vi "AWGCompileContinuousWave.vi"(2 "error in":errorcluster, 3 "ArbitraryWaveListMW":dbl[][](array[numeric]) caption="Arbitrary Waveform List") -> (0 "error out":errorcluster, 1 "array MW and RF":variant[](array[variant]))   [LabVIEW 2019]
panel:
  out "AWG array out":variant[](array[variant])
  in  "Timing cluster 2":T1
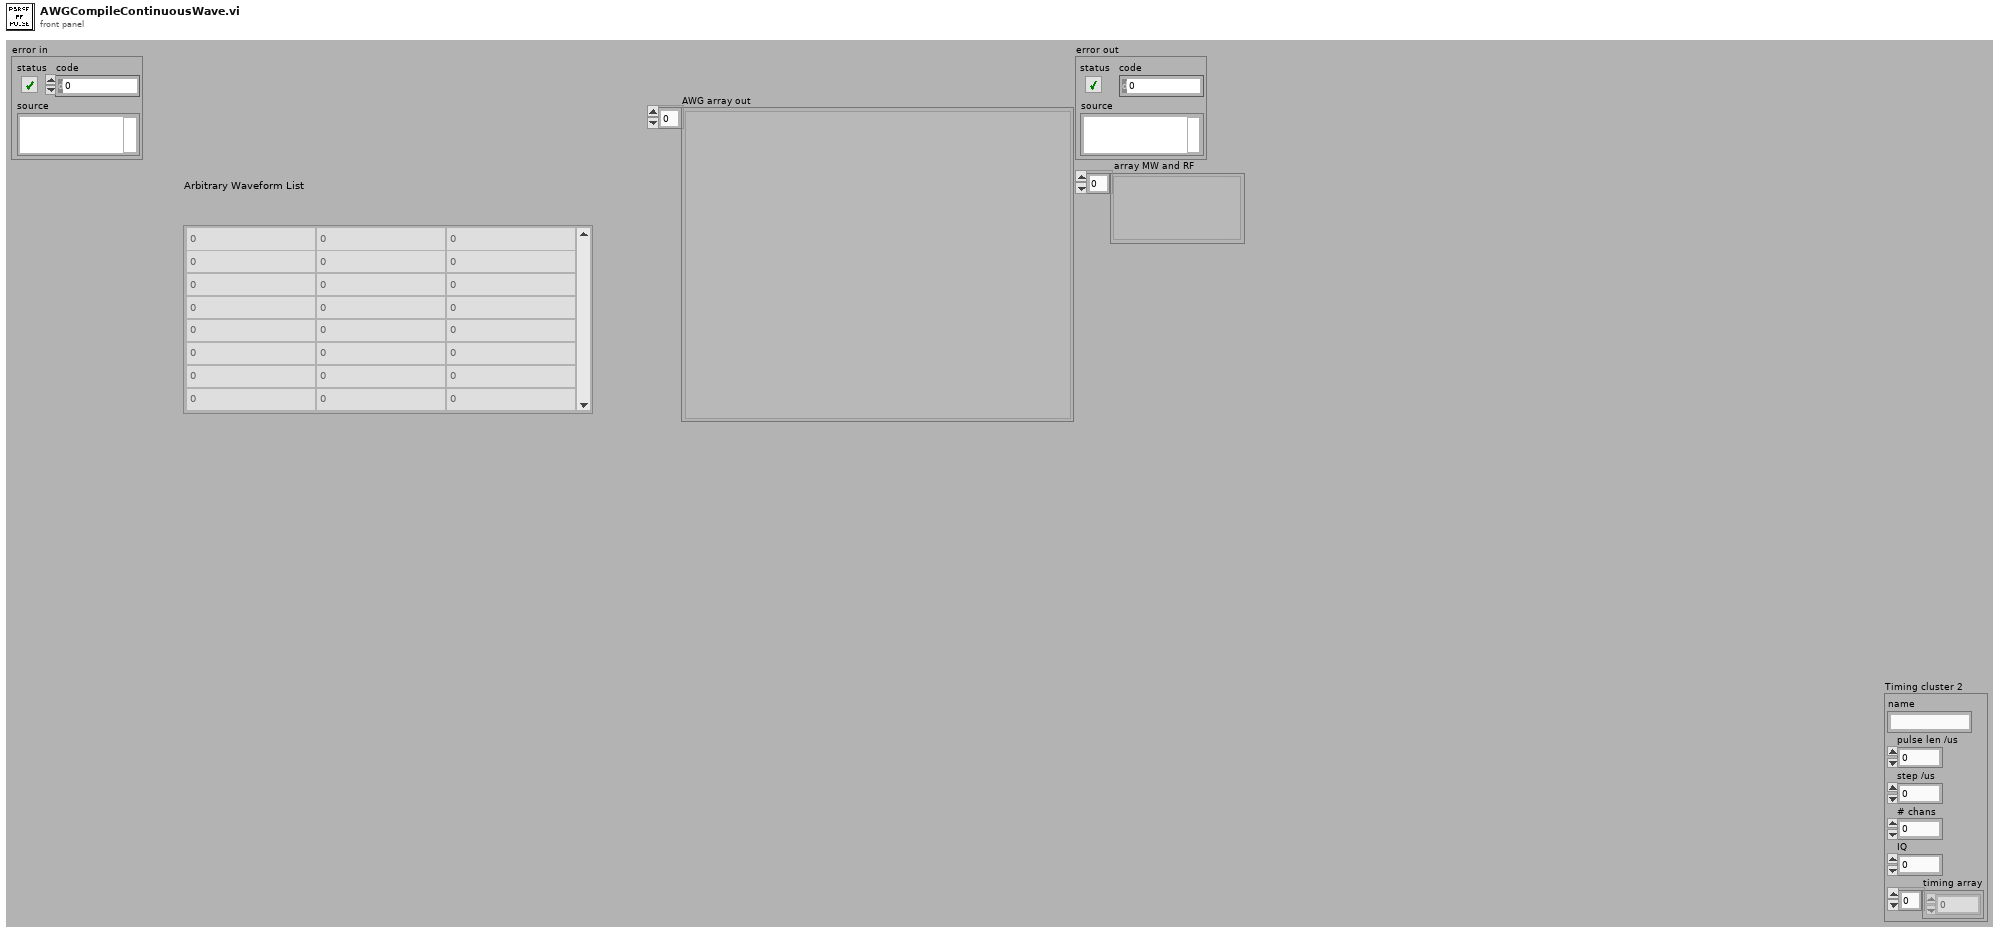
[diagram p1: front panel]
types:
  T1 = cluster{"name":string, "pulse len /us":dbl, "step /us":dbl, "# chans":i32, "IQ":i32, "timing array":dbl[]}
  T2 = cluster{"Timing cluster 2":cluster{"name":string, "pulse len /us":dbl, "step /us":dbl, "# chans":i32, "IQ":i32, "timing array":dbl[]}, "Channel cluster 2":cluster{"amp":dbl, "amp step":dbl, "channel array":dbl[]}[]}
  T3 = cluster{"amp":dbl, "amp step":dbl, "array type (2D Dbl)":dbl[]}
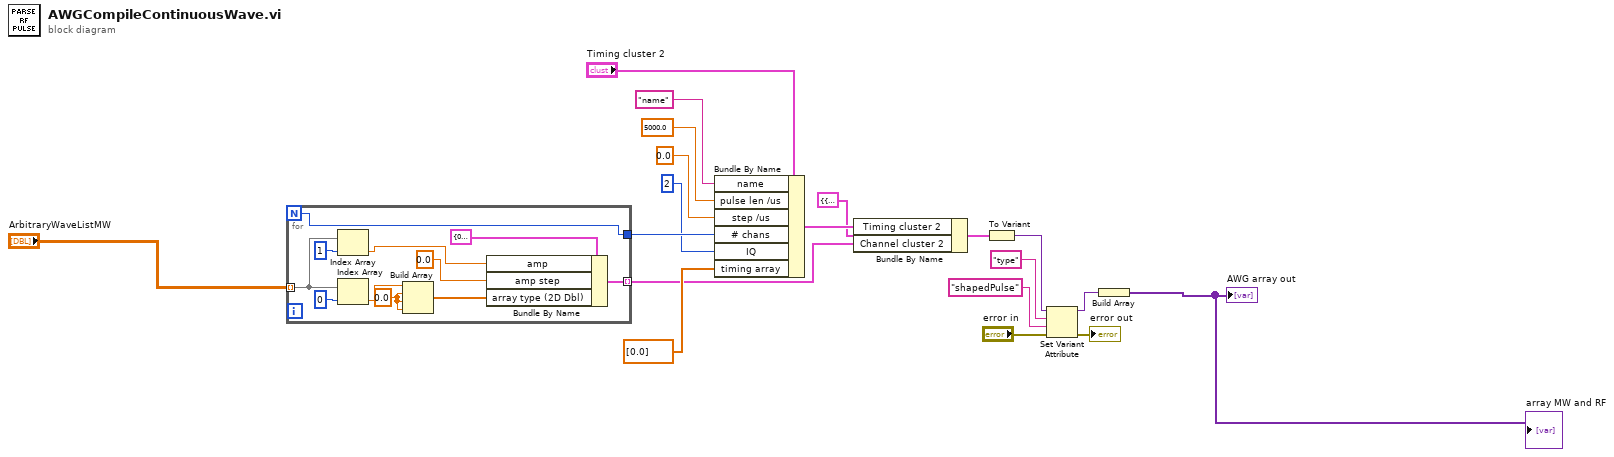
[diagram p0: block diagram]
diagram:
  n1 = for {
    N -> [w26]
    tunnel: "ArbitraryWaveListMW" -> [w23] mode=indexing
    tunnel: [w26] -> w9
    tunnel: [w20] -> w6 mode=indexing
    w25 = 0.0
    n2 = Index Array(array=w23, index=1) -> (element=w28:dbl)
    n3 = Index Array(array=w23, index=0) -> (element=w22:dbl)
    n4 = Build Array(w22, w25, w25, w25) -> (w21:dbl[])
    n5 = Bundle By Name(cluster=T3 {"amp"=0.0, "amp step"=0.0, "array type (2D Dbl)"=[]} ("freq cluster"), "amp"=w28, "amp step"=0.0, "array type (2D Dbl)"=w21) -> (w20:T3)
  }
  n6 = Bundle By Name(cluster="Timing cluster 2", "name"="name", "pulse len /us"=5000.0, "step /us"=0.0, "# chans"=w9, "IQ"=2, "timing array"=dbl[] [0.0]) -> (w19:T1)
  n7 = Bundle By Name(cluster=T2 {"Timing cluster 2"={"name"="", "pulse len /us"=0.0, "step /us"=0.0, "# chans"=0, "IQ"=0, "timing array"=[]}, "Channel cluster 2"=[]} ("RF pulse cluster"), "Timing cluster 2"=w19, "Channel cluster 2"=w6) -> (w17:T2)
  n8 = To Variant(anything=w17) -> (Variant=w16:variant)
  n9 = Set Variant Attribute(Variant=w16, name="type", value="shapedPulse", error in="error in") -> (Variant out=w5:variant, error out=→"error out":errorcluster)  [unwired: 1 out]
  n10 = Build Array(w5) -> (→"AWG array out" →"array MW and RF":variant[])
